vi "Go.vi"(9 "Timing Data":T1(array[cluster]), 10 "Control In":T2={"I-O.lvclass"=refnum, "Gantry"=refnum, "Dispenser"="COM1"}, 11 "C4 Dispense in":refnum<class "Iterative Dispense.lvclass">) -> (2 "Control Out":T2={"I-O.lvclass"=refnum, "Gantry"=refnum, "Dispenser"="COM1"}, 3 "C4 Dispense Out":refnum<class "Iterative Dispense.lvclass">)   [LabVIEW 2021, in "Iterative Dispense.lvclass"]
uses:
  Iterative Dispense.lvclass
  C:/Users/HEP/Documents/GitHub/Gantry/UCSB-Gantry-HEP-main/Classes/Routine/Dispense/Dispense.lvclass
  Controller/Controllers.ctl
  Controller/I-O/I-O.lvclass
  C:/Program Files (x86)/Aerotech/A3200/LabVIEW/2010/Bin/Aerotech.A3200.dll
  Program Files (x86)/Aerotech/A3200/LabVIEW/2010/Bin/Aerotech.A3200.dll
  Iterative Dispense.lvclass/Iterative Dispense.ctl
  Controller/Motion/A3200/A3200.lvclass
  Controller/Dispenser/Dispenser.lvclass
  Controller/Motion/Motion.lvclass
  Controller/Controller.lvclass
panel:
  out "error out":errorcluster
  in  "error in (no error)":errorcluster
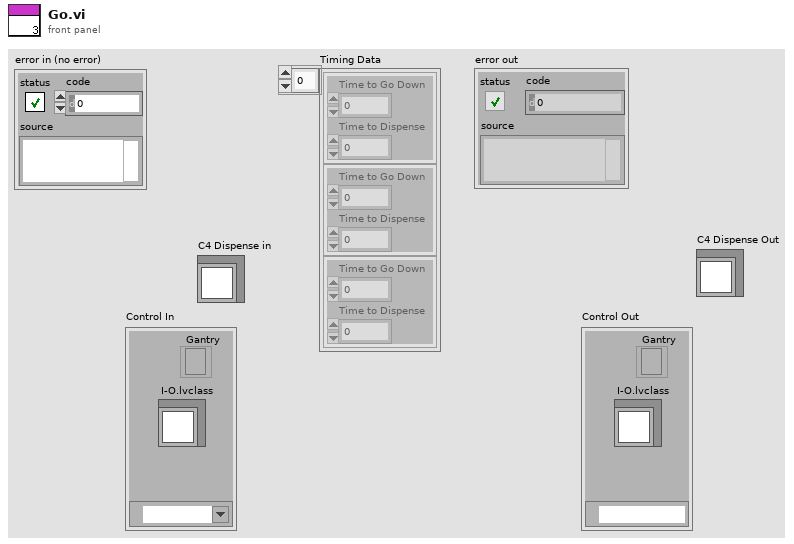
[diagram p1: front panel]
types:
  T1 = cluster{"Time to Go Down":i32, "Time to Dispense":i32}[]
  T2 = typedef "Controller.lvclass/Controllers.ctl" = cluster{"I-O.lvclass":refnum<class "I-O.lvclass">, "Gantry":refnum<k24>, "Dispenser":refnum<visa-resource-name>}
  T3 = typedef "Iterative Dispense.lvclass/Glue Step Enum.ctl" = enum16{"Baseplate to Kapton", "Kapton to Sensor"}
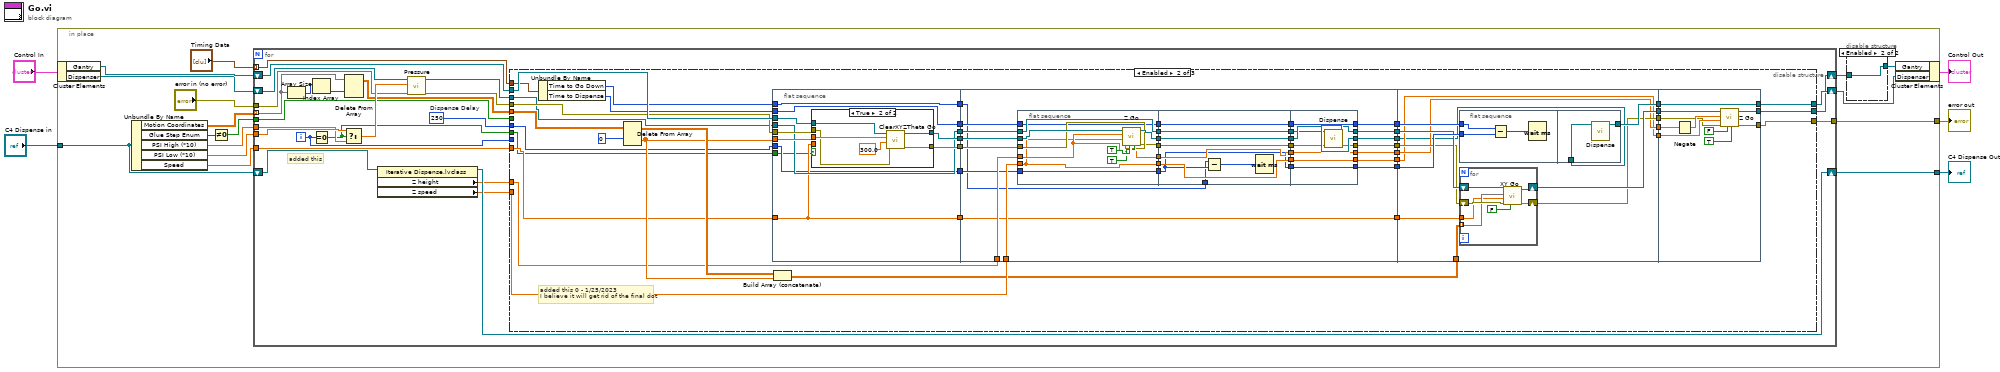
[diagram p0: block diagram]
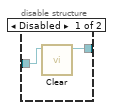
[diagram p2: hidden frame]
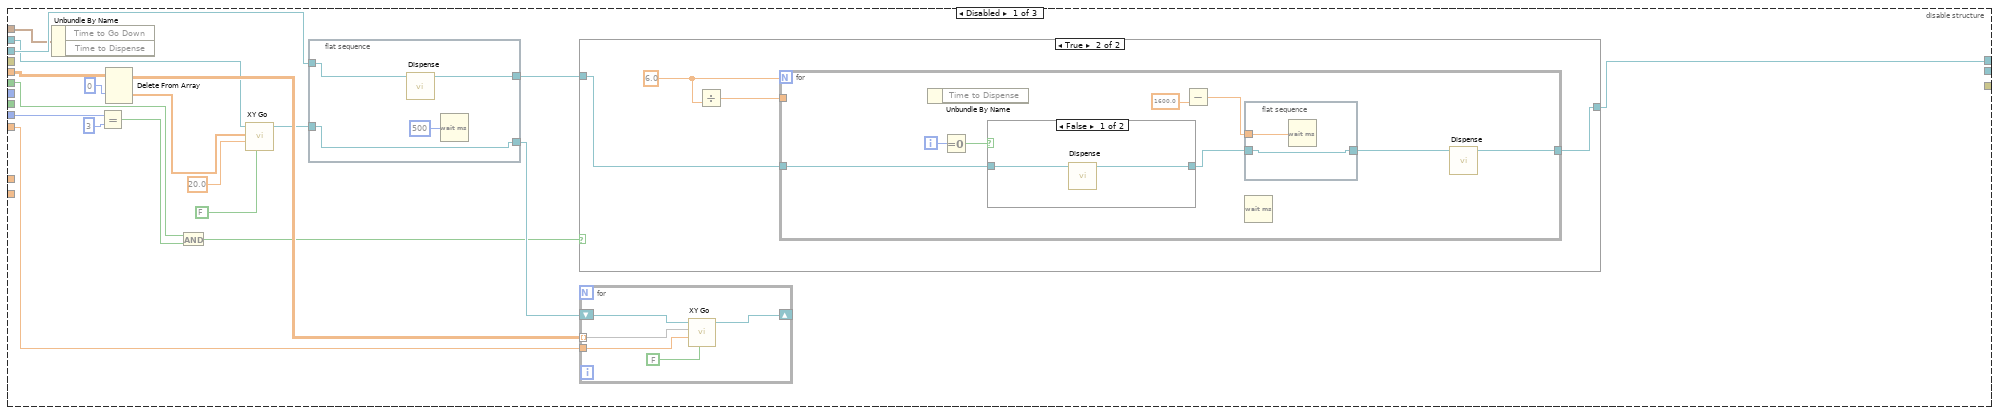
[diagram p3: hidden frame]
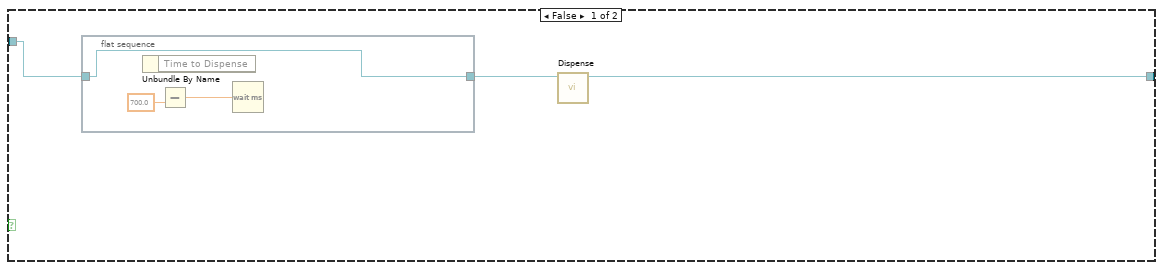
[diagram p4: hidden frame]
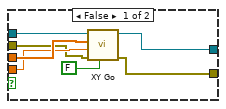
[diagram p6: hidden frame]
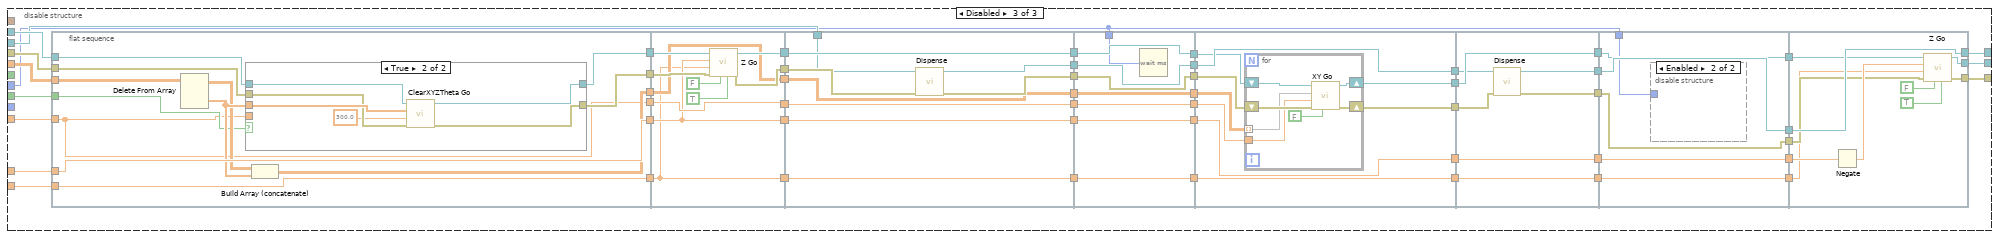
[diagram p7: hidden frame]
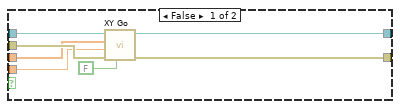
[diagram p8: hidden frame]
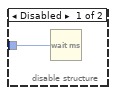
[diagram p9: hidden frame]
diagram:
  n1 = in-place {
    in-place-border: "C4 Dispense in" -> [w9]
    in-place-border: [w10] -> w2
    in-place-border: [w7] -> w1
    n2 = in-place-cluster #1("Control In") -> ("Gantry"=w15:refnum<k24>, "Dispenser"=w13:refnum<visa-resource-name>)
    n3 = Unbundle By Name(w9) -> ("Motion Coordinates"=w17:dbl[][][], "Glue Step Enum"=w16:T3, "PSI High (*10)"=w20:dbl, "PSI Low (*10)"=w19:dbl, "Speed"=w18:dbl)
    n4 = Not Equal To 0?(x=w16) -> (x != 0?=w21:bool)
    n5 = for {
      tunnel: w17 -> [w27] mode=indexing
      tunnel: w21 -> [w30]
      tunnel: w18 -> [w48]
      tunnel: w19 -> [w47]
      tunnel: w20 -> [w46]
      shift-right: [w32] -> w12
      shift-left: w15 -> [w44]
      shift-right: [w49] -> w14
      shift-left: w13 -> [w43]
      tunnel: "error in (no error)" -> [w40]
      shift-right: [w38] -> w10
      shift-left: w9 -> [w39]
      tunnel: [w34] -> w7
      tunnel: "Timing Data" -> [w31] mode=indexing
      i -> [w29]
      w35 = 250  # Dispense Delay
      # "added this"
      # "Executes C4 Symmetric Motion"
      n6 = Array Size(array=w27) -> (size(s)=w28:i32[])
      n7 = Index Array(array=w28) -> (element=w25:i32)  [unwired: 1 in]
      n8 = Equal To 0?(x=w29) -> (x = 0?=w33:bool)
      n9 = Select(t=w47, s=w33, f=w46) -> (s? t:f=w45:dbl)
      n10 = Delete From Array(array=w27, index (row)=w25) -> (array with subset deleted=w26:dbl[][])  [unwired: 2 in, 1 out]
      n11 = property class="Iterative Dispense.lvclass"(reference=w39) -> (reference out=w38:refnum<class "Iterative Dispense.lvclass">, "Z height"=w37:dbl, "Z speed"=w36:dbl)  [unwired: 1 in, 1 out]
      n12 = call "Pressure.vi"("error in (no error)"=w40, "Pressure"=w45, "VISA resource name"=w43) -> ("error out"=w41:errorcluster, "VISA resource name out"=w42:refnum<visa-resource-name>)  [unwired: 7 in]
      n13 = disable-structure shown="Enabled" {
        disable-tunnel: [w68 w113 w290] -> w49
        disable-tunnel: w26 -> [w67 w125 w292]
        disable-tunnel: w48 -> [w62 w122 w309]
        disable-tunnel: w42 -> [w61 w120 w291]
        disable-tunnel: w44 -> [w60 w127 w294]
        disable-tunnel: w41 -> [_ w121 w293]
        disable-tunnel: w37 -> [_ w118 w296]
        disable-tunnel: w36 -> [_ w117 w297]
        disable-tunnel: w35 -> [_ w109 w260]
        disable-tunnel: [_ w112 w289] -> w34
        disable-tunnel: w33 -> [_ w102 w295]
        disable-tunnel: [_ w126 w257] -> w32
        disable-tunnel: w31 -> [w55 w111 _]
        disable-tunnel: w30 -> [w54 _ _]
        disable-tunnel: w29 -> [w53 _ _]
        frame Disabled {
          n14 = Unbundle By Name(w55) -> ()  [unwired: 2 out]
          n15 = Equal?(x=w53, y=3) -> (x = y?=w51:bool)
          n16 = Delete From Array(array=w67, index (row)=0) -> (deleted portion=w58:dbl[], array with subset deleted=w65:dbl[][])  [unwired: 2 in]
          n17 = And(x=w54, y=w51) -> (x .and. y?=w50:bool)
          n18 = call "XY Go.vi"("return immediately"=FALSE, "Speed"=20.0 ("speed"), "XY In"=w58, "Gantry In"=w60) -> ("Gantry Out"=w59:refnum<k24>)  [unwired: 5 in, 2 out]
          n19 = flat-sequence {
            tunnel: w61 -> [w92]
            tunnel: w59 -> [w94]
            tunnel: [w94] -> w64
            tunnel: [w93] -> w63
            frame #0 {
              n20 = call "Dispense.vi"("Dispenser In"=w92) -> ("Dispenser Out"=w93:refnum<visa-resource-name>)  [unwired: 9 in, 1 out]
              n21 = Wait (ms)(milliseconds to wait=u32 500) -> ()  [unwired: 1 out]
            }
          }
          n22 = case shown="True" w50 {
            tunnel: w63 -> [w71 w77]
            tunnel: [w70 w76] -> w68
            frame False {
              n23 = flat-sequence {
                tunnel: w71 -> [w72]
                tunnel: [w72] -> w69
                frame #0 {
                  n24 = Unbundle By Name() -> ()  [unwired: 1 in, 1 out]
                  n25 = Subtract(y=700.0) -> (x-y=w74:dbl)  [unwired: 1 in]
                  n26 = Wait (ms)(milliseconds to wait=w74) -> ()  [unwired: 1 out]
                }
              }
              n27 = call "Dispense.vi"("Dispenser In"=w69) -> ("Dispenser Out"=w70:refnum<visa-resource-name>)  [unwired: 9 in, 1 out]
            }
            frame True {
              w75 = 6.0 ("y")
              # "Leaves Space for Silver Epoxy"
              n28 = Divide(y=w75) -> (x/y=w78:dbl)  [unwired: 1 in]
              n29 = for {
                N: w75 -> [_]
                tunnel: w78 -> [_]
                tunnel: w77 -> [w84]
                tunnel: [w80] -> w76
                i -> [w82]
                n30 = Unbundle By Name() -> ()  [unwired: 1 in, 1 out]
                n31 = Equal To 0?(x=w82) -> (x = 0?=w81:bool)
                n32 = case shown="False" w81 {
                  tunnel: w84 -> [w87 w89]
                  tunnel: [w88 w89] -> w83
                  frame False {
                    n33 = call "Dispense.vi"("Dispenser In"=w87) -> ("Dispenser Out"=w88:refnum<visa-resource-name>)  [unwired: 9 in, 1 out]
                  }
                  frame True {
                  }
                }
                n34 = Subtract(y=1600.0) -> (x-y=w85:dbl)  [unwired: 1 in]
                n35 = flat-sequence {
                  tunnel: w85 -> [w91]
                  tunnel: w83 -> [w90]
                  tunnel: [w90] -> w79
                  frame #0 {
                    n36 = Wait (ms)(milliseconds to wait=w91) -> ()  [unwired: 1 out]
                  }
                }
                n37 = Wait (ms)() -> ()  [unwired: 1 in, 1 out]
                n38 = call "Dispense.vi"("Dispenser In"=w79) -> ("Dispenser Out"=w80:refnum<visa-resource-name>)  [unwired: 9 in, 1 out]
              }
            }
          }
          n39 = for {
            tunnel: w62 -> [w97]
            tunnel: w65 -> [w98] mode=indexing
            shift-right: [w99] -> _
            shift-left: w64 -> [w100]
            n40 = call "XY Go.vi"("return immediately"=FALSE, "Speed"=w97, "XY In"=w98, "Gantry In"=w100) -> ("Gantry Out"=w99:refnum<k24>)  [unwired: 5 in, 2 out]
          }
        }
        frame Enabled {
          # "added this 0 - 1/25/2023\nI believe it will get rid of the final dot"
          n41 = Unbundle By Name(w111) -> ("Time to Go Down"=w106:i32, "Time to Dispense"=w104:i32)
          n42 = Delete From Array "Delete From Array"(array=w125, index (row)=0) -> (deleted portion=w123:dbl[], array with subset deleted=w124:dbl[][])  [unwired: 2 in]
          n43 = flat-sequence {
            tunnel: w127 -> [w150]
            tunnel: [w149] -> w139
            tunnel: [w146] -> w138
            tunnel: w123 -> [w148]
            tunnel: w122 -> [w144]
            tunnel: w121 -> [w147]
            tunnel: w120 -> [w145]
            tunnel: [w145] -> w119
            tunnel: [w144] -> w115
            tunnel: [w143] -> w110
            tunnel: w109 -> [w143]
            tunnel: [w142] -> w107
            tunnel: w106 -> [w142]
            tunnel: [w141] -> w105
            tunnel: w104 -> [w141]
            tunnel: w102 -> [w140]
            tunnel: w139 -> [w192]
            tunnel: [w193] -> w137
            tunnel: [w191] -> w136
            tunnel: w138 -> [w190]
            tunnel: [w188] -> w135
            tunnel: [w187] -> w134
            tunnel: [w186] -> w133
            tunnel: w119 -> [w189]
            tunnel: w118 -> [w185]
            tunnel: w117 -> [w184]
            tunnel: w115 -> [w183]
            tunnel: [w183] -> w114
            tunnel: w110 -> [w182]
            tunnel: [w181] -> w108
            tunnel: w107 -> [w164]
            tunnel: w105 -> [w180]
            tunnel: [w179] -> w103
            tunnel: w137 -> [w223]
            tunnel: [w234] -> w132
            tunnel: w136 -> [w231]
            tunnel: [w227] -> w131
            tunnel: [w225] -> w130
            tunnel: w135 -> [w225]
            tunnel: [w224] -> w129
            tunnel: w134 -> [w224]
            tunnel: w133 -> [w230]
            tunnel: [w226] -> w128
            tunnel: w116 -> [w229]
            tunnel: w114 -> [w228]
            tunnel: w108 -> [w233]
            tunnel: w103 -> [w232]
            tunnel: [w256] -> w126
            tunnel: w132 -> [w255]
            tunnel: [w255] -> w113
            tunnel: w131 -> [w254]
            tunnel: [w253] -> w112
            tunnel: w130 -> [w252]
            tunnel: w129 -> [w250]
            tunnel: w128 -> [w247]
            frame #0 {
              n44 = case shown="True" w140 {
                tunnel: w150 -> [w157 w163]
                tunnel: [w156 w162] -> w149
                tunnel: [w155 w161] -> w146
                tunnel: w148 -> [w153 w160]
                tunnel: w144 -> [w152 _]
                tunnel: w147 -> [w151 w159]
                frame False {
                  n45 = call "XY Go.vi"("return immediately"=FALSE, "error in (no error)"=w151, "Speed"=w152, "XY In"=w153, "Gantry In"=w157) -> ("error out"=w155:errorcluster, "Gantry Out"=w156:refnum<k24>)  [unwired: 4 in, 1 out]
                }
                frame True {
                  n46 = call "ClearXYZTheta Go.vi"("error in (no error)"=w159, "Speed"=300.0, "XYZTheta In"=w160, "Gantry In"=w163) -> ("error out"=w161:errorcluster, "Gantry Out"=w162:refnum<k24>)  [unwired: 5 in, 1 out]
                }
              }
            }
            frame #1 {
              n47 = flat-sequence {
                tunnel: w192 -> [w204]
                tunnel: [w202] -> w178
                tunnel: w190 -> [w199]
                tunnel: [w201] -> w176
                tunnel: w189 -> [w201]
                tunnel: [w194] -> w174
                tunnel: [w198] -> w172
                tunnel: w185 -> [w195]
                tunnel: w184 -> [w194]
                tunnel: [w197] -> w170
                tunnel: w182 -> [w197]
                tunnel: w180 -> [w196]
                tunnel: [w196] -> w168
                tunnel: [w195] -> w166
                tunnel: w178 -> [w213]
                tunnel: [w213] -> w177
                tunnel: w176 -> [w212]
                tunnel: [w212] -> w175
                tunnel: w174 -> [w211]
                tunnel: [w211] -> w173
                tunnel: w172 -> [w210]
                tunnel: [w210] -> w171
                tunnel: w170 -> [w207]
                tunnel: [w207] -> w169
                tunnel: w168 -> [w209]
                tunnel: [w209] -> w167
                tunnel: w166 -> [w208]
                tunnel: [w208] -> w165
                tunnel: w164 -> [w206]
                tunnel: [w222] -> w193
                tunnel: w177 -> [w221]
                tunnel: [w221] -> w191
                tunnel: w175 -> [w220]
                tunnel: [w219] -> w188
                tunnel: [w218] -> w187
                tunnel: w173 -> [w218]
                tunnel: w171 -> [w217]
                tunnel: [w216] -> w186
                tunnel: [w215] -> w181
                tunnel: w169 -> [w215]
                tunnel: [w214] -> w179
                tunnel: w167 -> [w214]
                tunnel: w165 -> [w219]
                frame #0 {
                  n48 = call "Z Go.vi"("Increment"=TRUE, "Return Immediately"=TRUE, "error in (no error)"=w199, "Speed In"=w194, "Position In"=w195, "Gantry In"=w204) -> ("error out"=w198:errorcluster, "Gantry Out"=w202:refnum<k24>)  [unwired: 2 in, 2 out]
                }
                frame #1 {
                  n49 = Subtract(x=w206, y=w207) -> (x-y=w205:i32)
                  n50 = Wait (ms)(milliseconds to wait=w205) -> ()  [unwired: 1 out]
                }
                frame #2 {
                  n51 = call "Dispense.vi"("error in (no error)"=w217, "Dispenser In"=w220) -> ("error out"=w216:errorcluster, "Dispenser Out"=w222:refnum<visa-resource-name>)  [unwired: 8 in]
                }
              }
            }
            frame #2 {
              n52 = flat-sequence {
                tunnel: w233 -> [w244]
                tunnel: w232 -> [w243]
                tunnel: [w246] -> w234
                tunnel: w223 -> [w245]
                frame #0 {
                  n53 = Subtract(x=w243, y=w244) -> (x-y=w242:i32)
                  n54 = Wait (ms)(milliseconds to wait=w242) -> ()  [unwired: 1 out]
                }
                frame #1 {
                  n55 = call "Dispense.vi"("Dispenser In"=w245) -> ("Dispenser Out"=w246:refnum<visa-resource-name>)  [unwired: 9 in, 1 out]
                }
              }
              n56 = for {
                shift-right: [w239] -> w227
                shift-left: w231 -> [w240]
                shift-right: [w237] -> w226
                shift-left: w230 -> [w238]
                tunnel: w229 -> [w236] mode=indexing
                tunnel: w228 -> [w235]
                n57 = call "XY Go.vi"("return immediately"=FALSE, "error in (no error)"=w238, "Speed"=w235, "XY In"=w236, "Gantry In"=w240) -> ("error out"=w237:errorcluster, "Gantry Out"=w239:refnum<k24>)  [unwired: 4 in, 1 out]
              }
            }
            frame #3 {
              n58 = Negate(x=w252) -> (-x=w251:dbl)
              n59 = call "Z Go.vi"("Increment"=TRUE, "Return Immediately"=FALSE, "error in (no error)"=w247, "Speed In"=w250, "Position In"=w251, "Gantry In"=w254) -> ("error out"=w253:errorcluster, "Gantry Out"=w256:refnum<k24>)  [unwired: 2 in, 2 out]
            }
          }
          n60 = Build Array (concatenate)(w124, w123) -> (w116:dbl[][])
        }
        frame Disabled {
          n61 = flat-sequence {
            tunnel: w297 -> [w320]
            tunnel: w296 -> [w321]
            tunnel: [w313] -> w308
            tunnel: [w312] -> w307
            tunnel: [w321] -> w306
            tunnel: [w320] -> w305
            tunnel: w295 -> [w317]
            tunnel: w294 -> [w316]
            tunnel: w293 -> [w315]
            tunnel: w309 -> [w310]
            tunnel: w292 -> [w314]
            tunnel: [w311] -> w288
            tunnel: [w310] -> w286
            tunnel: [w342] -> w304
            tunnel: [w339] -> w303
            tunnel: w308 -> [w344]
            tunnel: w307 -> [w340]
            tunnel: w306 -> [w336]
            tunnel: w305 -> [w335]
            tunnel: w288 -> [w338]
            tunnel: [w338] -> w287
            tunnel: w286 -> [w337]
            tunnel: [w337] -> w285
            tunnel: [w336] -> w259
            tunnel: [w335] -> w258
            tunnel: w304 -> [w352]
            tunnel: w303 -> [w349]
            tunnel: w291 -> [w347]
            tunnel: [w353] -> w284
            tunnel: [w352] -> w282
            tunnel: [w351] -> w280
            tunnel: [w350] -> w278
            tunnel: [w348] -> w276
            tunnel: w287 -> [w346]
            tunnel: [w346] -> w274
            tunnel: w285 -> [w345]
            tunnel: [w345] -> w272
            tunnel: w259 -> [w351]
            tunnel: w258 -> [w350]
            tunnel: w284 -> [w361]
            tunnel: [w361] -> w283
            tunnel: w282 -> [w360]
            tunnel: [w360] -> w281
            tunnel: w280 -> [w359]
            tunnel: [w359] -> w279
            tunnel: w278 -> [w358]
            tunnel: [w358] -> w277
            tunnel: w276 -> [w357]
            tunnel: [w357] -> w275
            tunnel: w274 -> [w356]
            tunnel: [w356] -> w273
            tunnel: w272 -> [w355]
            tunnel: [w355] -> w271
            tunnel: w260 -> [w354]
            tunnel: w283 -> [w370]
            tunnel: w281 -> [w367]
            tunnel: w279 -> [w369]
            tunnel: w277 -> [w368]
            tunnel: w275 -> [w365]
            tunnel: [w370] -> w302
            tunnel: [w366] -> w301
            tunnel: [w369] -> w300
            tunnel: [w368] -> w299
            tunnel: [w364] -> w298
            tunnel: w273 -> [w363]
            tunnel: w271 -> [w362]
            tunnel: w302 -> [w379]
            tunnel: w301 -> [w384]
            tunnel: w300 -> [w383]
            tunnel: w299 -> [w382]
            tunnel: w298 -> [w381]
            tunnel: [w378] -> w270
            tunnel: [w384] -> w268
            tunnel: [w383] -> w266
            tunnel: [w382] -> w264
            tunnel: [w380] -> w262
            tunnel: w270 -> [w390]
            tunnel: [w390] -> w269
            tunnel: w268 -> [w389]
            tunnel: [w389] -> w267
            tunnel: w266 -> [w388]
            tunnel: [w388] -> w265
            tunnel: w264 -> [w387]
            tunnel: [w387] -> w263
            tunnel: w262 -> [w386]
            tunnel: [w386] -> w261
            tunnel: w260 -> [w385]
            tunnel: [w396] -> w257
            tunnel: [w401] -> w290
            tunnel: w269 -> [w401]
            tunnel: w267 -> [w397]
            tunnel: w265 -> [w393]
            tunnel: w263 -> [w392]
            tunnel: w261 -> [w395]
            tunnel: [w394] -> w289
            frame #0 {
              n62 = Delete From Array(array=w314) -> (deleted portion=w319:dbl[], array with subset deleted=w318:dbl[][])  [unwired: 3 in]
              n63 = case shown="True" w317 {
                tunnel: [w327 w334] -> w313
                tunnel: [w326 w333] -> w312
                tunnel: w319 -> [w322 w332]
                tunnel: w316 -> [w328 w331]
                tunnel: w315 -> [w324 w330]
                tunnel: w310 -> [w323 _]
                frame False {
                  n64 = call "XY Go.vi"("return immediately"=FALSE, "error in (no error)"=w324, "Speed"=w323, "XY In"=w322, "Gantry In"=w328) -> ("error out"=w326:errorcluster, "Gantry Out"=w327:refnum<k24>)  [unwired: 4 in, 1 out]
                }
                frame True {
                  n65 = call "ClearXYZTheta Go.vi"("error in (no error)"=w330, "Speed"=300.0, "XYZTheta In"=w332, "Gantry In"=w331) -> ("error out"=w333:errorcluster, "Gantry Out"=w334:refnum<k24>)  [unwired: 5 in, 1 out]
                }
              }
              n66 = Build Array (concatenate)(w318, w319) -> (w311:dbl[][])
            }
            frame #1 {
              n67 = call "Z Go.vi"("Increment"=TRUE, "Return Immediately"=FALSE, "error in (no error)"=w340, "Speed In"=w335, "Position In"=w336, "Gantry In"=w344) -> ("error out"=w339:errorcluster, "Gantry Out"=w342:refnum<k24>)  [unwired: 2 in, 2 out]
            }
            frame #2 {
              n68 = call "Dispense.vi"("error in (no error)"=w349, "Dispenser In"=w347) -> ("error out"=w348:errorcluster, "Dispenser Out"=w353:refnum<visa-resource-name>)  [unwired: 8 in]
            }
            frame #3 {
              n69 = Wait (ms)(milliseconds to wait=w354) -> ()  [unwired: 1 out]
            }
            frame #4 {
              n70 = for {
                shift-right: [w375] -> w366
                shift-left: w367 -> [w376]
                shift-right: [w373] -> w364
                shift-left: w365 -> [w374]
                tunnel: w363 -> [w372] mode=indexing
                tunnel: w362 -> [w371]
                n71 = call "XY Go.vi"("return immediately"=FALSE, "error in (no error)"=w374, "Speed"=w371, "XY In"=w372, "Gantry In"=w376) -> ("error out"=w373:errorcluster, "Gantry Out"=w375:refnum<k24>)  [unwired: 4 in, 1 out]
              }
            }
            frame #5 {
              n72 = call "Dispense.vi"("error in (no error)"=w381, "Dispenser In"=w379) -> ("error out"=w380:errorcluster, "Dispenser Out"=w378:refnum<visa-resource-name>)  [unwired: 8 in]
            }
            frame #6 {
              n73 = disable-structure shown="Enabled" {
                disable-tunnel: w385 -> [w391 _]
                frame Disabled {
                  n74 = Wait (ms)(milliseconds to wait=w391) -> ()  [unwired: 1 out]
                }
                frame Enabled {
                }
              }
            }
            frame #7 {
              n75 = Negate(x=w393) -> (-x=w400:dbl)
              n76 = call "Z Go.vi"("Increment"=TRUE, "Return Immediately"=FALSE, "error in (no error)"=w395, "Speed In"=w392, "Position In"=w400, "Gantry In"=w397) -> ("error out"=w394:errorcluster, "Gantry Out"=w396:refnum<k24>)  [unwired: 2 in, 2 out]
            }
          }
        }
      }
    }
    n77 = disable-structure shown="Enabled" {
      disable-tunnel: w12 -> [w23 w24]
      disable-tunnel: [w22 w24] -> w11
      frame Disabled {
        n78 = call "Clear.vi"("Gantry In"=w23) -> ("Gantry Out"=w22:refnum<k24>)  [unwired: 9 in, 1 out]
      }
      frame Enabled {
      }
    }
    n79 = in-place-cluster #1("Gantry"=w11, "Dispenser"=w14) -> (→"Control Out":T2)
  }
  "C4 Dispense Out" <- w2
  "error out" <- w1
